vi "regu-sce-to-cmd.vi"(11 "regulate-pannel":T1) -> (3 "regulate-cmd":string[](array[string]))   [LabVIEW 2019]
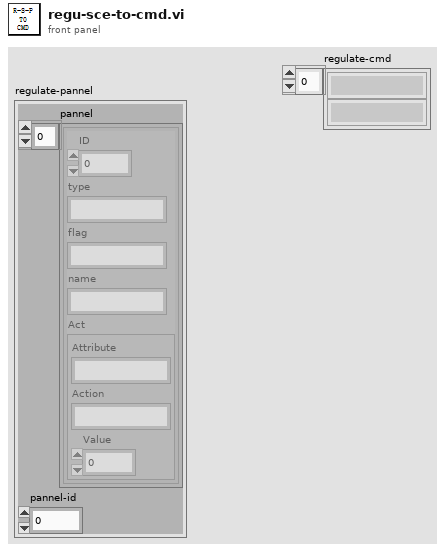
[diagram p1: front panel]
types:
  T1 = cluster{"pannel":cluster{"ID":u8, "type":string, "flag":string, "name":string, "Act":cluster{"Attribute":string, "Action":string, "Value":dbl}}[], "pannel-id":dbl}
  T2 = cluster{"ID":u8, "type":string, "flag":string, "name":string, "Act":cluster{"Attribute":string, "Action":string, "Value":dbl}}[]
  T3 = cluster{"ID":u8, "type":string, "flag":string, "name":string, "Act":cluster{"Attribute":string, "Action":string, "Value":dbl}}
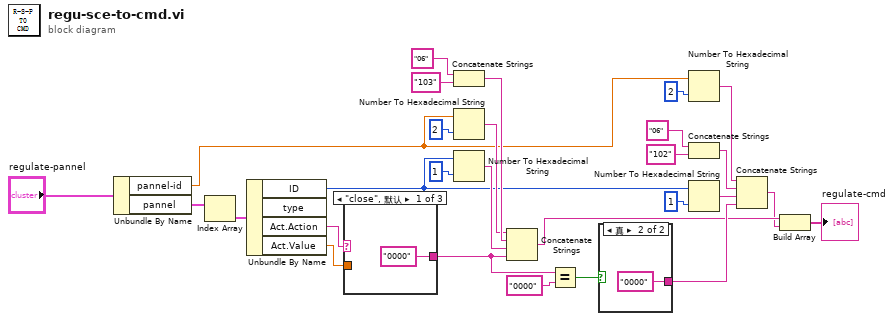
[diagram p0: block diagram]
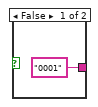
[diagram p2: hidden frame]
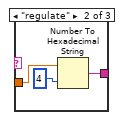
[diagram p3: hidden frame]
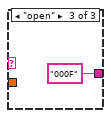
[diagram p4: hidden frame]
diagram:
  n1 = Unbundle By Name("regulate-pannel") -> ("pannel-id"=w6:dbl, "pannel"=w28:T2)
  n2 = Index Array(array=w28) -> (element=w27:T3)  [unwired: 1 in]
  n3 = Unbundle By Name(w27) -> ("ID"=w5:u8, "Act.Action"=w18:string, "Act.Value"=w17:dbl)  [unwired: 1 out]
  n4 = case shown="\"close\", 默认" w18 {
    tunnel: w17 -> [_ w31 _]
    tunnel: ["0000" w30 "000F"] -> w16
    frame "close", Default {
    }
    frame "regulate" {
      n5 = Number To Hexadecimal String(1:i16 4 ("宽度(-)"), 2:w31) -> (0:w30:string)
    }
    frame "open" {
    }
  }
  n6 = Concatenate Strings("06" ("字符串"), "103" ("字符串")) -> (w25:string)
  n7 = Number To Hexadecimal String(1:i16 2 ("宽度(-)"), 2:w6) -> (0:w23:string)
  n8 = Number To Hexadecimal String(1:i16 1 ("宽度(-)"), 2:w5) -> (0:w21:string)
  n9 = Concatenate Strings(w23, w25, w21, w16) -> (w3:string)
  n10 = Equal?(x=w16, y="0000") -> (x = y?=w14:bool)
  n11 = case shown="真" w14 {
    tunnel: ["0001" "0000"] -> w4
    frame False {
    }
    frame True {
    }
  }
  n12 = Number To Hexadecimal String(1:i16 2 ("宽度(-)"), 2:w6) -> (0:w10:string)
  n13 = Concatenate Strings("06" ("字符串"), "102" ("字符串")) -> (w8:string)
  n14 = Number To Hexadecimal String(1:i16 1 ("宽度(-)"), 2:w5) -> (0:w12:string)
  n15 = Concatenate Strings(w10, w8, w12, w4) -> (w2:string)
  n16 = Build Array(w3, w2) -> (→"regulate-cmd":string[])
